vi "generate cylinder knock settings.vi"(10 "Convert Val":dbl, 11 "Cylinder Knock Configuration":T2(array[cluster])) -> (2 "cylinder knock inputs":T1[](array[typedef]), 3 "Cylinder Knock Settings":T3[](array[typedef]))   [LabVIEW 2015]
uses:
  IP Source/Knock Sensor/Cylinder Settings.ctl
  IP Source/Knock Sensor/Cylinder Input.ctl
  IP Source/Knock Sensor/Knock Sensor.lvlib
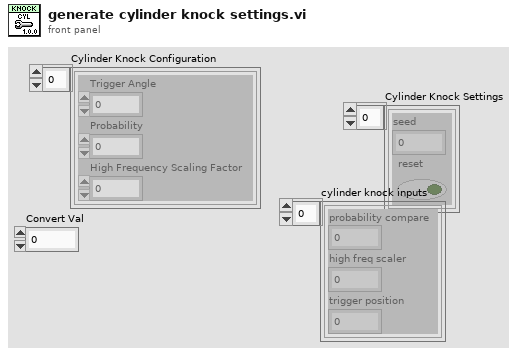
[diagram p1: front panel]
types:
  T1 = typedef "Engine Simulation Toolkit.lvlib/Knock Sensor.lvlib/Cylinder Input.ctl" = cluster{"probability compare":u16, "high freq scaler":fxp<+,10,0>, "trigger position":u16}
  T2 = cluster{"Trigger Angle":dbl, "Probability":dbl, "High Frequency Scaling Factor":dbl}[]
  T3 = typedef "Engine Simulation Toolkit.lvlib/Knock Sensor.lvlib/Cylinder Settings.ctl" = cluster{"seed":u16, "reset":bool}
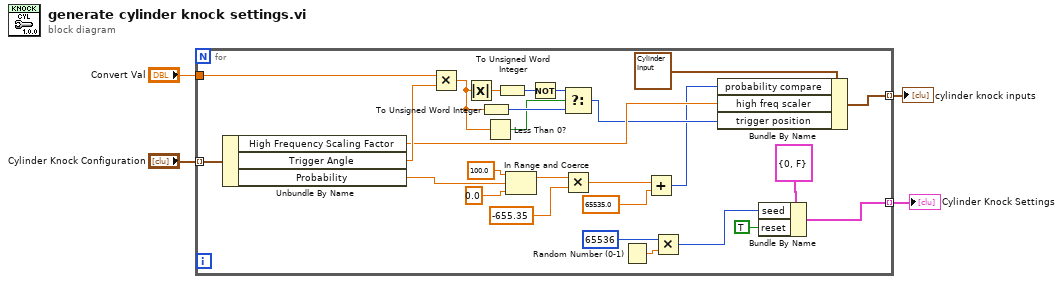
[diagram p0: block diagram]
diagram:
  n1 = for {
    tunnel: "Cylinder Knock Configuration" -> [w30] mode=indexing
    tunnel: [w26] -> w4 mode=indexing
    tunnel: "Convert Val" -> [w18]
    tunnel: [w16] -> w1 mode=indexing
    n2 = Unbundle By Name(w30) -> ("High Frequency Scaling Factor"=w15:dbl, "Trigger Angle"=w19:dbl, "Probability"=w11:dbl)
    n3 = Multiply(x=w18, y=w19) -> (x*y=w20:dbl)
    n4 = Absolute Value(x=w20) -> (abs(x)=w24:dbl)
    n5 = To Unsigned Word Integer(number=w20) -> (unsigned 16bit integer=w22:u16)
    n6 = Less Than 0?(x=w20) -> (x < 0?=w21:bool)
    n7 = To Unsigned Word Integer(number=w24) -> (unsigned 16bit integer=w25:u16)
    n8 = In Range and Coerce(upper limit=100.0, x=w11, lower limit=0.0) -> (coerced(x)=w7:dbl)  [unwired: 1 out]
    n9 = Not(x=w25) -> (.not. x?=w23:u16)
    n10 = Select(t=w23, s=w21, f=w22) -> (s? t:f=w14:u16)
    n11 = Multiply(x=w7, y=-655.35) -> (x*y=w9:dbl)
    n12 = Random Number (0-1)() -> (number: 0 to 1=w29:dbl)
    n13 = Add(x=w9, y=65535.0) -> (x+y=w6:u16)
    n14 = Multiply(x=u32 65536 ("seed"), y=w29) -> (x*y=w27:u16)
    n15 = Bundle By Name(cluster=T1 {"probability compare"=0, "high freq scaler"=0.0, "trigger position"=0} ("Cylinder Knock Configuration"), "probability compare"=w6, "high freq scaler"=w15, "trigger position"=w14) -> (w16:T1)
    n16 = Bundle By Name(cluster=T3 {"seed"=0, "reset"=FALSE} ("Cylinder Knock Configuration"), "seed"=w27, "reset"=TRUE) -> (w26:T3)
  }
  "Cylinder Knock Settings" <- w4
  "cylinder knock inputs" <- w1
